vi "Send Start Trigger.vi"(8 "error in (no error)":errorcluster, 11 "VISA resource name":refnum<visa-resource-name>) -> (0 "error out":errorcluster, 3 "VISA resource name out":refnum<visa-resource-name>)   [LabVIEW 2024, in "Micron Optics sm130.lvlib"]
doc: "Initiates a software start trigger in Software triggering mode. This VI can also be used to simulate a hardware trigger start when the module is set to hardware triggering mode."
uses:
  Micron Optics sm130.lvlib
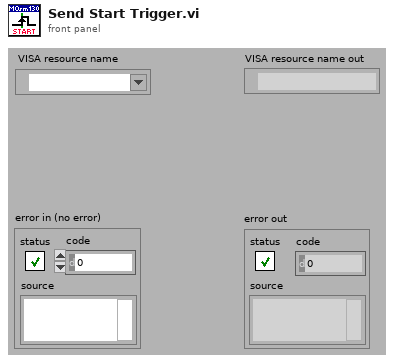
[diagram p1: front panel]
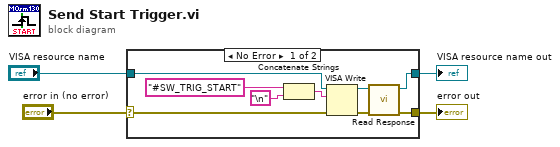
[diagram p0: block diagram]
diagram:
  n1 = case shown="No Error" "error in (no error)" {
    selector: "error in (no error)" -> [w5 w14]
    tunnel: "VISA resource name" -> [w10 w15]
    tunnel: [w7 w15] -> w3
    tunnel: [w6 w14] -> w2
    frame No Error {
      n2 = Concatenate Strings("#SW_TRIG_START" ("write buffer"), "\n") -> (w13:string)
      n3 = VISA Write(VISA resource name=w10, write buffer=w13, error in (no error)=w5) -> (VISA resource name out=w9:refnum<visa-resource-name>, error out=w8:errorcluster)  [unwired: 1 out]
      n4 = call "Read Response.vi"("error in (no error)"=w8, "VISA resource name"=w9) -> ("error out"=w6:errorcluster, "VISA resource name out"=w7:refnum<visa-resource-name>)  [unwired: 7 in, 1 out]
    }
    frame Error {
    }
  }
  "VISA resource name out" <- w3
  "error out" <- w2
